vi "Set Graph Properties.vi"(8 "error out 2":errorcluster, 10 "Selected Variables":string[][](array[string]), 11 "Reference Array":refnum<vi>[](array[refnum])) -> (0 "error out":errorcluster, 3 "Legend rows":i32)   [LabVIEW 2013]
doc: "This vi sets the properties of xy graph\n[Input]\n1. Plot names\n2. xy graph\n3. Error in\n[output]\nError out"
panel:
  in  "Color Array":u32[](array[colorbox])=[16711680, 23220, 16711907, 32639, 16746240, 6618880, 3381759, 11748095, 16774233]
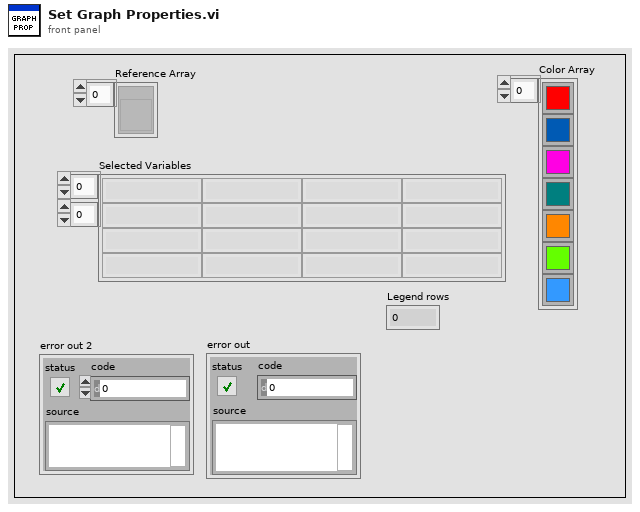
[diagram p1: front panel]
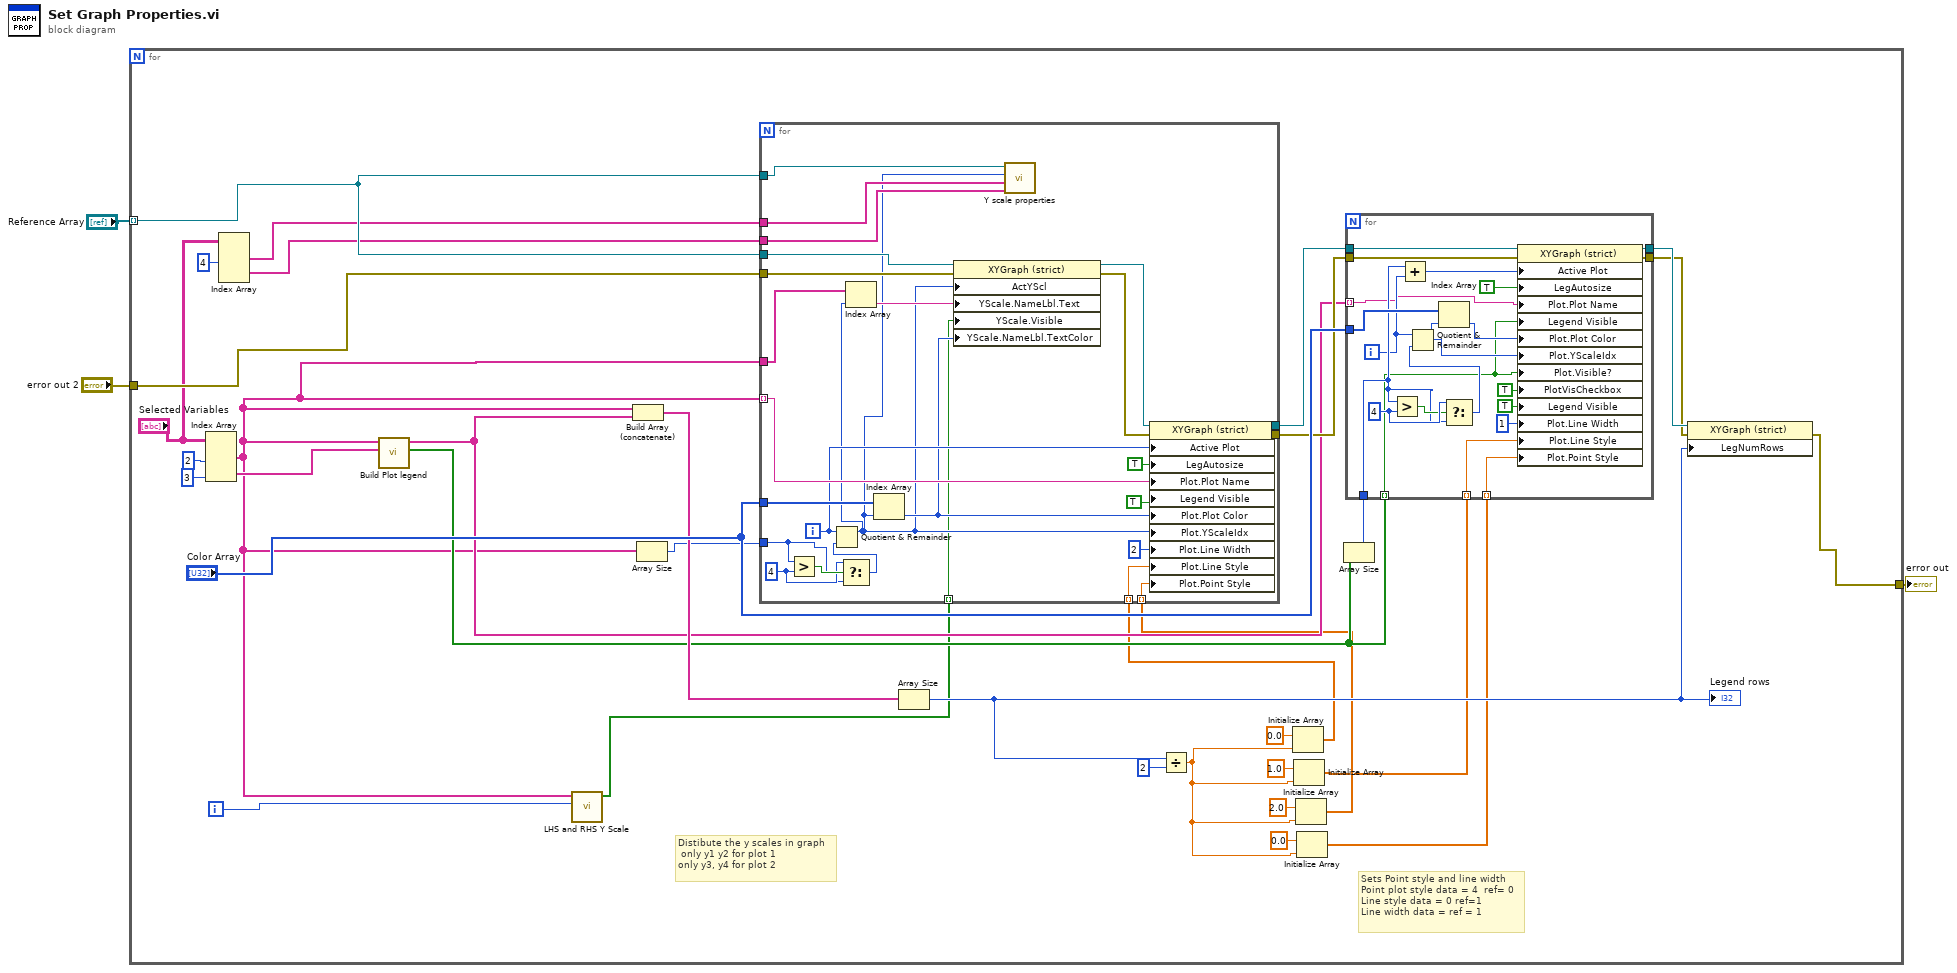
[diagram p0: block diagram]
diagram:
  n1 = for {
    tunnel: [w36] -> w3
    tunnel: "Reference Array" -> [w35] mode=indexing
    tunnel: "error out 2" -> [w34]
    i -> [w26]
    # "Sets Point style and line width\nPoint plot style data = 4  ref= 0\nLine style data = 0 ref=1\nLine width data = ref = 1"
    # "Distibute the y scales in graph\n only y1 y2 for plot 1\nonly y3, y4 for plot 2"
    n2 = Index Array(array="Selected Variables", index (col) #1=2 ("disabled index (col)"), index (col) #2=3 ("index (col)")) -> (element #1=w16:string[], element #2=w31:string[])  [unwired: 2 in]
    n3 = Index Array(array="Selected Variables", index (col) #1=4 ("disabled index (col)")) -> (element #1=w28:string[], element #2=w27:string[])  [unwired: 3 in]
    n4 = call "Build Plot legend.vi"("Reference Values"=w31, "Display Names"=w16) -> ("Array"=w18:bool[], "Plot legend Names"=w20:string[])  [unwired: 8 in]
    n5 = call "LHS and RHS Y Scale.vi"("Numeric"=w26, "Selected Variables"=w16) -> ("Array"=w4:bool[])  [unwired: 9 in]
    n6 = Build Array (concatenate)(w16, w20) -> (w25:string[])
    n7 = Array Size(array=w16) -> (size(s)=w19:i32)
    n8 = Array Size(array=w25) -> (size(s)=w15:i32)
    "Legend rows" <- w15
    n9 = Divide(x=w15, y=2) -> (x/y=w9:dbl)
    n10 = Initialize Array(0.0 ("element"), w9) -> (w7:dbl[])
    n11 = Initialize Array(1.0 ("element"), w9) -> (w6:dbl[])
    n12 = Initialize Array(2.0 ("element"), w9) -> (w8:dbl[])
    n13 = for {
      tunnel: w16 -> [w83] mode=indexing
      tunnel: w35 -> [w69]
      tunnel: [w84] -> w24
      tunnel: w19 -> [w71]
      tunnel: "Color Array" -> [w82]
      tunnel: w34 -> [w79]
      tunnel: [w77] -> w22
      tunnel: w16 -> [w76]
      tunnel: w28 -> [w67]
      tunnel: w27 -> [w66]
      tunnel: w35 -> [w68]
      tunnel: w4 -> [w62] mode=indexing
      tunnel: w7 -> [w60] mode=indexing
      tunnel: w8 -> [w59] mode=indexing
      i -> [w74]
      w72 = 4 ("y")
      n14 = Greater?(x=w71, y=w72) -> (0:w73:bool)
      n15 = Select(t=w72, s=w73, f=w71) -> (s? t:f=w70:i32)
      n16 = Quotient & Remainder(x=w74, y=w70) -> (x-y*floor(x/y)=w64:i32)  [unwired: 1 out]
      n17 = Index Array(array=w76, index=w64) -> (element=w75:string)
      n18 = Index Array(array=w82, index=w64) -> (element=w65:u32)
      n19 = property class="XYGraph (strict)"(reference=w69, error in=w79, "ActYScl"=w64, "YScale.NameLbl.Text"=w75, "YScale.Visible"=w62, "YScale.NameLbl.TextColor"=w65) -> (reference out=w80:refnum<vi>, error out=w78:errorcluster)
      n20 = call "Y scale properties.vi"("Min"=w66, "Max"=w67, "Active index"=w64, "XYGraph in"=w68) -> ()  [unwired: 8 in]
      n21 = property class="XYGraph (strict)"(reference=w80, error in=w78, "Active Plot"=w74, "LegAutosize"=TRUE ("Legend:Autosize"), "Plot.Plot Name"=w83, "Legend Visible"=TRUE ("Legend:Visible"), "Plot.Plot Color"=w65, "Plot.YScaleIdx"=w64, "Plot.Line Width"=u8 2, "Plot.Line Style"=w60, "Plot.Point Style"=w59) -> (reference out=w84:refnum<vi>, error out=w77:errorcluster)
    }
    n22 = Initialize Array(0.0 ("element"), w9) -> (w5:dbl[])
    n23 = Array Size(array=w18) -> (size(s)=w17:i32)
    n24 = for {
      tunnel: w24 -> [w58]
      tunnel: [w57] -> w23
      tunnel: w20 -> [w41] mode=indexing
      tunnel: "Color Array" -> [w56]
      tunnel: [w55] -> w21
      tunnel: w22 -> [w51]
      tunnel: w17 -> [w50]
      tunnel: w18 -> [w45] mode=indexing
      tunnel: w6 -> [w39] mode=indexing
      tunnel: w5 -> [w38] mode=indexing
      i -> [w47]
      w54 = 4 ("y")
      n25 = Greater?(x=w50, y=w54) -> (0:w53:bool)
      n26 = Add(x=w50, y=w47) -> (x+y=w48:i32)
      n27 = Select(t=w54, s=w53, f=w50) -> (s? t:f=w52:i32)
      n28 = Quotient & Remainder(x=w47, y=w52) -> (x-y*floor(x/y)=w46:i32)  [unwired: 1 out]
      n29 = Index Array(array=w56, index=w46) -> (element=w49:u32)
      n30 = property class="XYGraph (strict)"(reference=w58, error in=w51, "Active Plot"=w48, "LegAutosize"=TRUE ("Legend:Autosize"), "Plot.Plot Name"=w41, "Legend Visible"=w45, "Plot.Plot Color"=w49, "Plot.YScaleIdx"=w46, "Plot.Visible?"=w45, "PlotVisCheckbox"=TRUE ("Legend:Plot Visibility Checkbox Visible"), "Legend Visible"=TRUE ("Legend:Visible"), "Plot.Line Width"=u8 1, "Plot.Line Style"=w39, "Plot.Point Style"=w38) -> (reference out=w57:refnum<vi>, error out=w55:errorcluster)
    }
    n31 = property class="XYGraph (strict)"(reference=w23, error in=w21, "LegNumRows"=w15) -> (error out=w36:errorcluster)  [unwired: 1 out]
  }
  "error out" <- w3
